vi "sequence util_makeloop.vi"(8 "error in":errorcluster, 9 "Item Names IN":string[](array[string])=["----------    AH Bridge: Save GPIB address   ", "Write to VISA, GPIB::27::INSTR, FILE STORE GPIB USERPON", "----------    LakeShore 340 controller: change heater power (0-5, 0: off)  ", "Write to VISA, GPIB::12::INSTR, RANGE 0", "----------    Scheduled T-control for the He3 system   ", "Wait for 12 hour", "Set Temperature LS336 ( GPIB0::12::INSTR ) 45 K at 0 K/min, Output 1", "Wait for 60 s", "Wait for Temperature Less than 1.8 K Sensor C of LS336 ( GPIB0::14::INSTR ) Timeout 30 min", "Wait for 60 min", "Set Temperature LS336 ( GPIB0::12::INSTR ) 0.1 K at 0 K/min, Output 1", "----------    Motor control (use Instrumet:Set:MotorControl command structure)  ", "Set MotorControl ( BLM ) 12345 0.2", "Wait for VI value localhost, BLM_ManualControl.vi, BLM Position, Within, 12345, 10 min", "Wait for 10 s", "END SEQUENCE"]) -> (0 "error out":errorcluster, 1 "Item Names out":string[](array[string]), 3 "sequence out":string, 11 "sequence in":string="0: ----------    AH Bridge: Save GPIB address   \n1: Write to VISA, GPIB::27::INSTR, FILE STORE GPIB USERPON\n2: ----------    LakeShore 340 controller: change heater power (0-5, 0: off)  \n3: Write to VISA, GPIB::12::INSTR, RANGE 0\n4: ----------    Scheduled T-control for the He3 system   \n5: Wait for 12 hour\n6: Set Temperature LS336 ( GPIB0::12::INSTR ) 45 K at 0 K/min, Output 1\n7: Wait for 60 s\n8: Wait for Temperature Less than 1.8 K Sensor C of LS336 ( GPIB0::14::INSTR ) Timeout 30 min\n9: Wait for 60 min\n10: Set Temperature LS336 ( GPIB0::12::INSTR ) 0.1 K at 0 K/min, Output 1\n11: ----------    Motor control (use Instrumet:Set:MotorControl command structure)  \n12: Set MotorControl ( BLM ) 12345 0.2\n13: Wait for VI value localhost, BLM_ManualControl.vi, BLM Position, Within, 12345, 10 min\n14: Wait for 10 s\n15: END SEQUENCE")   [LabVIEW 2020]
panel:
  in  "valid?":bool
  out "extracted No.":dbl
  in  "Cancel":bool
  in  "Done":bool
  out "keyword":string
  in  "strings after the variable":string="INSTR )"
  in  "line # for the variable":u16=8
  in  "varialbe step":dbl=5.0 min=0.0
  in  "varialbe stop":dbl=10.0
  in  "varialbe start":dbl=45.0
  in  "strings before the variable":string="INSTR )"
  in  "line # for loop end":u16=9
  in  "line # for loop begin":u16=5
  # "(1)"
  # "keyword: a string that includes the variable. Only a number in the keyword will be identified \nas variable. \nTry different set of 'before' and 'after' strings to find the desired keyword."
  # "(3)"
  # "(2)"
  # "Make a loop: a block of sequence repeats itself while a variable inside the block changes \nits value (determined by start, stop, step).\n\n(1) Define a block to be repeated.\n(2) Identify a keyword that contains the changing variable.\n          i) select the line # that contains the variable.\n         ii) assign strings 'before' and 'after' to extract the keyword\n(3) Confirm the extracted No. and keyward are valid.\n(4) Set the loop condition (start. stop, step)\n\nSequence out window will show resulting loop sequence real time."
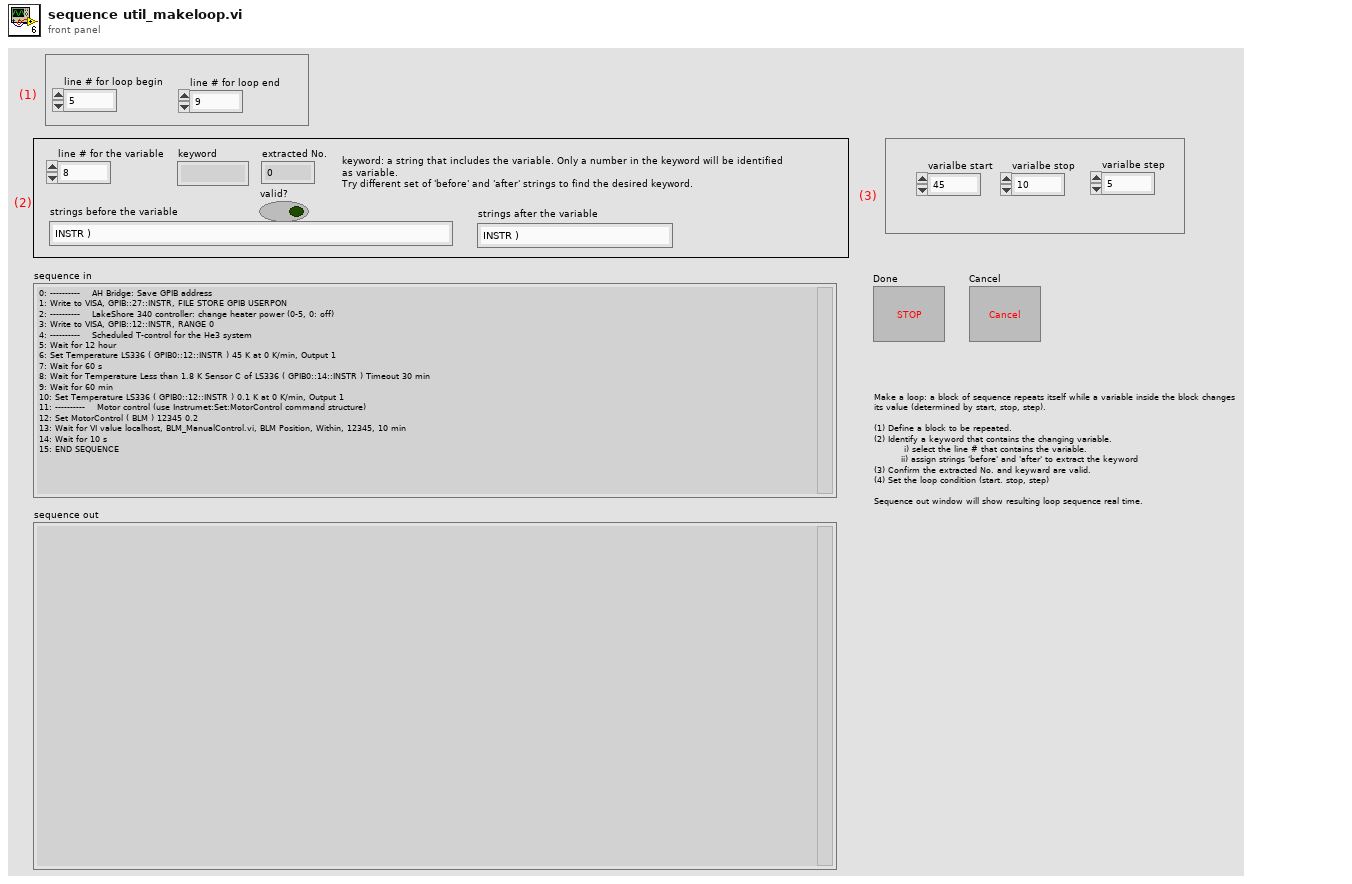
[diagram p1: front panel]
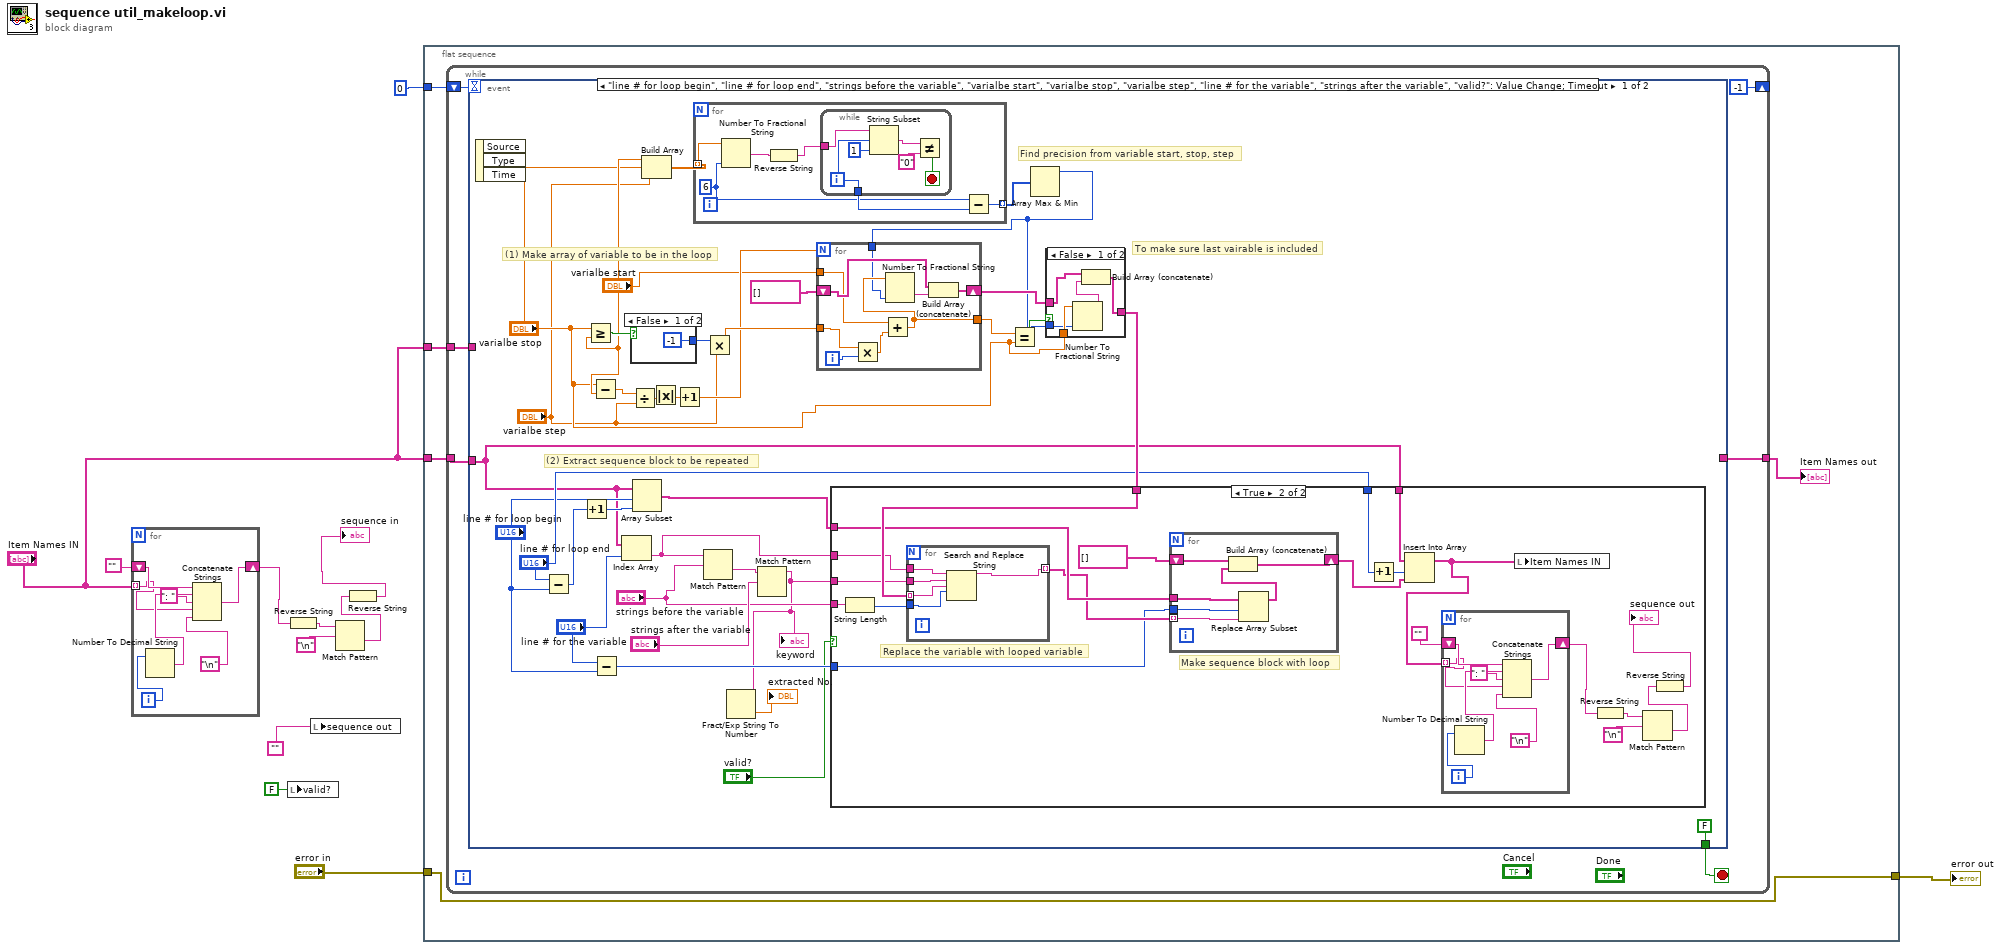
[diagram p0: block diagram]
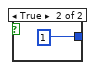
[diagram p4: hidden frame]
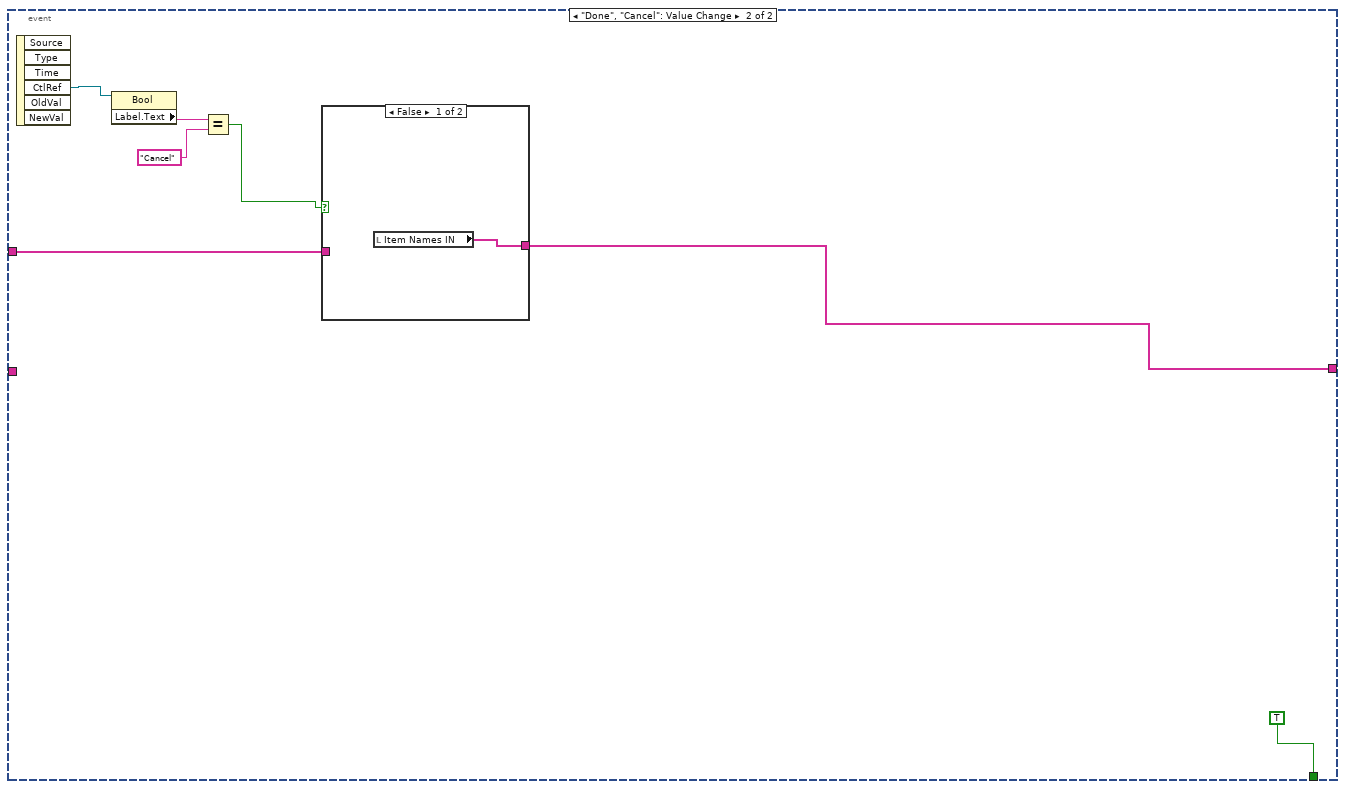
[diagram p5: hidden frame]
diagram:
  n1 = for {
    shift-right: [w18] -> w12
    shift-left: "" -> [w19]
    tunnel: "Item Names IN" -> [w14] mode=indexing
    i -> [w17]
    n2 = Number To Decimal String(number=w17) -> (decimal integer string=w16:string)  [unwired: 1 in]
    n3 = Concatenate Strings(w19, w16, ": " ("string"), w14, "\n") -> (w18:string)
  }
  n4 = local write "valid?"(FALSE ("valid?")) -> ()
  n5 = Reverse String(1:w12) -> (0:w11:string)
  n6 = local write "sequence out"("") -> ()
  n7 = Match Pattern(string=w11, regular expression="\n") -> (after substring=w9:string)  [unwired: 1 in, 3 out]
  n8 = Reverse String(1:w9) -> (0:→"sequence in":string)
  n9 = flat-sequence {
    tunnel: [w23] -> w5
    tunnel: "Item Names IN" -> [w24]
    tunnel: "error in" -> [w23]
    tunnel: "Item Names IN" -> [w21]
    tunnel: 0 -> [w20]
    frame #0 {
      n10 = while {
        tunnel: w21 -> [w29]
        tunnel: w24 -> [w27]
        tunnel: [w28] -> w22
        shift-right: [-1] -> _
        shift-left: w20 -> [w25]
        stop <- w30 stop-if-true
        n11 = event shown="[0] \"line # for loop begin\", \"line # for loop end\", \"strings before the variable\", \"varialbe start\", \"varialbe stop\", \"varialbe step\", \"line # for the variable\", \"strings after the variable\", \"valid?\": Value Change;  Timeout" {
          selector: _ -> [_ _]
          dyn-events: _ -> [_ _]
          timeout: w25 -> [_ _]
          tunnel: [FALSE TRUE] -> w30
          tunnel: [_ w132] -> w28
          tunnel: w29 -> [_ w133]
          tunnel: w27 -> [w34 _]
          event "line # for loop begin", "line # for loop end", "strings before the variable", "varialbe start", "varialbe stop", "varialbe step", "line # for the variable", "strings after the variable", "valid?": Value Change; Timeout {
            # "Find precision from variable start, stop, step"
            # "To make sure last vairable is included"
            # "(2) Extract sequence block to be repeated"
            # "(1) Make array of variable to be in the loop"
            n12 = event-data() -> ()  [unwired: 1 in, 3 out]
            n13 = Subtract(x="line # for loop end", y="line # for loop begin") -> (x-y=w64:u16)
            n14 = Increment(x=w64) -> (x+1=w63:u16)
            n15 = Greater Or Equal?(x="varialbe stop", y="varialbe start") -> (x >= y?=w53:bool)
            n16 = Subtract(x="varialbe stop", y="varialbe start") -> (x-y=w59:dbl)
            n17 = Subtract(x="line # for the variable", y="line # for loop begin") -> (x-y=w49:u16)
            n18 = Index Array(array=w34, index="line # for the variable") -> (element=w46:string)
            n19 = case shown="False" w53 {
              tunnel: [-1 1] -> w61
              frame False {
              }
              frame True {
              }
            }
            n20 = Divide(x=w59, y="varialbe step") -> (x/y=w58:dbl)
            n21 = Array Subset(array=w34, index="line # for loop begin", length=w63) -> (w55:string[])
            n22 = Build Array("varialbe start", "varialbe stop", "varialbe step") -> (w38:dbl[])
            n23 = Absolute Value(x=w58) -> (abs(x)=w57:dbl)
            n24 = Increment(x=w57) -> (x+1=w54:dbl)
            n25 = for {
              tunnel: w38 -> [w108] mode=indexing
              tunnel: [w103] -> w37 mode=indexing
              w104 = i16 6 ("precision (6)")
              n26 = Number To Fractional String(number=w108, precision (6)=w104) -> (F-format string=w107:string)  [unwired: 2 in]
              n27 = Reverse String(1:w107) -> (0:w106:string)
              n28 = while {
                tunnel: [w110] -> w105
                tunnel: w106 -> [w111]
                i -> [w110]
                stop <- w109 stop-if-true
                n29 = String Subset(string=w111, offset (0)=w110, length (rest)=1 ("length (rest)")) -> (substring=w113:string)
                n30 = Not Equal?(x=w113, y="0" ("substring")) -> (x != y?=w109:bool)
              }
              n31 = Subtract(x=w104, y=w105) -> (x-y=w103:i32)
            }
            n32 = Match Pattern(string=w46, regular expression="strings before the variable") -> (after substring=w48:string)  [unwired: 1 in, 3 out]
            n33 = Multiply(x=w61, y="varialbe step") -> (x*y=w60:dbl)
            n34 = Match Pattern(string=w48, regular expression="strings after the variable") -> (before substring=w33:string)  [unwired: 1 in, 3 out]
            "keyword" <- w33
            n35 = Fract/Exp String To Number(string=w33) -> (number=→"extracted No.":dbl)  [unwired: 3 in, 1 out]
            n36 = Array Max & Min(array=w37) -> (max value=w36:i32)  [unwired: 3 out]
            n37 = for {
              N: w54 -> [_]
              shift-right: [w128] -> w43
              shift-left: string[] [] -> [w127]
              tunnel: w60 -> [w124]
              tunnel: "varialbe start" -> [w126]
              tunnel: [w122] -> w44
              tunnel: w36 -> [w121]
              i -> [w125]
              n38 = Multiply(x=w124, y=w125) -> (x*y=w123:dbl)
              n39 = Add(x=w126, y=w123) -> (x+y=w122:dbl)
              n40 = Number To Fractional String(number=w122, precision (6)=w121) -> (F-format string=w129:string)  [unwired: 2 in]
              n41 = Build Array (concatenate)(w127, w129) -> (w128:string[])
            }
            n42 = Equal?(x=w44, y="varialbe stop") -> (x = y?=w42:bool)
            n43 = case shown="False" w42 {
              tunnel: [w117 w120] -> w56
              tunnel: w43 -> [w119 w120]
              tunnel: "varialbe stop" -> [w116 _]
              tunnel: w36 -> [w115 _]
              frame False {
                n44 = Number To Fractional String(number=w116, precision (6)=w115) -> (F-format string=w118:string)  [unwired: 2 in]
                n45 = Build Array (concatenate)(w119, w118) -> (w117:string[])
              }
              frame True {
              }
            }
            n46 = case shown="True" "valid?" {
              tunnel: w56 -> [_ w83]
              tunnel: w55 -> [_ w82]
              tunnel: "line # for loop end" -> [_ w72]
              tunnel: w49 -> [_ w71]
              tunnel: w46 -> [_ w70]
              tunnel: "strings before the variable" -> [_ w69]
              tunnel: w33 -> [_ w67]
              tunnel: w34 -> [_ w65]
              frame False {
              }
              frame True {
                # "Make sequence block with loop"
                # "Replace the variable with looped variable"
                n47 = String Length(string=w69) -> (length=w68:i32)
                n48 = for {
                  tunnel: w70 -> [w94]
                  tunnel: w67 -> [w96]
                  tunnel: w83 -> [w95] mode=indexing
                  tunnel: [w92] -> w81 mode=indexing
                  tunnel: w68 -> [w93]
                  n49 = Search and Replace String(input string=w94, search string=w96, replace string=w95, offset=w93) -> (result string=w92:string)  [unwired: 4 in, 3 out]
                }
                n50 = for {
                  shift-right: [w101] -> w80
                  shift-left: string[] [] -> [w102]
                  tunnel: w82 -> [w100]
                  tunnel: w71 -> [w99]
                  tunnel: w81 -> [w98] mode=indexing
                  n51 = Replace Array Subset(array=w100, new element=w98, index=w99) -> (w97:string[])
                  n52 = Build Array (concatenate)(w102, w97) -> (w101:string[])
                }
                n53 = Increment(x=w72) -> (x+1=w79:u16)
                n54 = Insert Into Array(array=w65, index=w79, new element=w80) -> (w66:string[])
                n55 = for {
                  shift-right: [w90] -> w78
                  shift-left: "" -> [w91]
                  tunnel: w66 -> [w86] mode=indexing
                  i -> [w89]
                  n56 = Number To Decimal String(number=w89) -> (decimal integer string=w88:string)  [unwired: 1 in]
                  n57 = Concatenate Strings(w91, w88, ": " ("string"), w86, "\n") -> (w90:string)
                }
                n58 = local write "Item Names IN"(w66) -> ()
                n59 = Reverse String(1:w78) -> (0:w77:string)
                n60 = Match Pattern(string=w77, regular expression="\n") -> (after substring=w75:string)  [unwired: 1 in, 3 out]
                n61 = Reverse String(1:w75) -> (0:→"sequence out":string)
              }
            }
          }
          event "Done", "Cancel": Value Change {
            n62 = event-data() -> ("CtlRef"=w137:refnum<vi>)  [unwired: 1 in, 5 out]
            n63 = property class="Bool"(reference=w137) -> ("Label.Text"=w136:string)  [unwired: 1 in, 2 out]
            n64 = Equal?(x=w136, y="Cancel") -> (x = y?=w134:bool)
            n65 = case shown="False" w134 {
              tunnel: [w139 w140] -> w132
              tunnel: w133 -> [_ w140]
              frame False {
                n66 = local read "Item Names IN"() -> (w139:string[])
              }
              frame True {
              }
            }
          }
        }
      }
      "Item Names out" <- w22
    }
  }
  "error out" <- w5
